vi "Untitled 2.vi"() -> ()   [LabVIEW 2019]
panel:
  out "output 1":timestamp
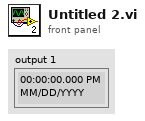
[diagram p1: front panel]
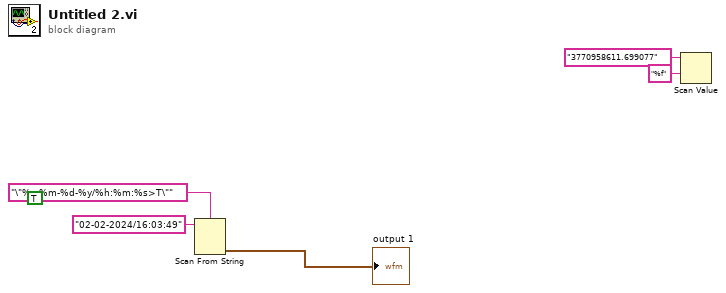
[diagram p0: block diagram]
diagram:
  (unwired) TRUE ("UTC format")
  n1 = Scan From String(format string="\"%<%m-%d-%y/%h:%m:%s>T\"", input string="02-02-2024/16:03:49") -> (output 1=→"output 1":timestamp)  [unwired: 3 in, 3 out]
  n2 = Scan Value(string="3770958611.699077", format string="%f") -> ()  [unwired: 1 in, 2 out]
